vi "movtreeitems.vi"(2 "error out 2":errorcluster, 3 "Array":T1(array[cluster]), 4 "String":string, 5 "Tree 2":refnum<vi>) -> (0 "error out":errorcluster, 1 "Tree":refnum<vi>)   [LabVIEW 2010]
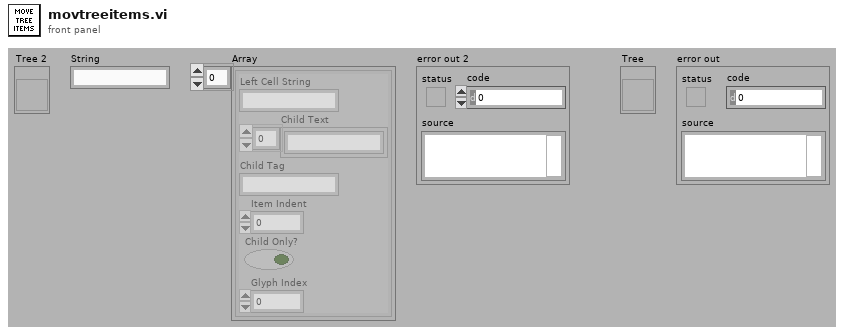
[diagram p1: front panel]
types:
  T1 = cluster{"Left Cell String":string, "Child Text":string[], "Child Tag":string, "Item Indent":i32, "Child Only?":bool, "Glyph Index":i32}[]
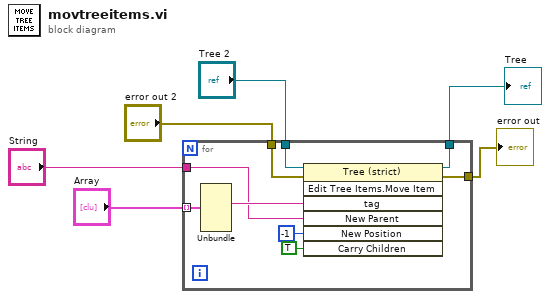
[diagram p0: block diagram]
diagram:
  n1 = for {
    tunnel: "Tree 2" -> [w15]
    tunnel: "error out 2" -> [w14]
    tunnel: [w13] -> w3
    tunnel: [w12] -> w4
    tunnel: "Array" -> [w11] mode=indexing
    tunnel: "String" -> [w9]
    n2 = Unbundle(w11) -> ("Child Tag"=w10:string)  [unwired: 5 out]
    n3 = invoke on="Invoke Node" class="Tree (strict)" method="Edit Tree Items.Move Item"(reference=w15, error in=w14, "tag"=w10, "New Parent"=w9, "New Position"=-1, "Carry Children"=TRUE ("Carry Children?")) -> (reference out=w13:refnum<vi>, error out=w12:errorcluster)  [unwired: 1 in, 5 out]
  }
  "error out" <- w4
  "Tree" <- w3
